vi "適應性控制_線上學習_V8(實際控制).vi"() -> ()   [LabVIEW 2010]
uses:
  <vilib>/DAQmx/read.llb/DAQmx Read (Analog 1D Wfm NChan NSamp).vi
  <vilib>/DAQmx/write.llb/DAQmx Write (Analog DBL 1Chan 1Samp).vi
  <vilib>/DAQmx/create/channels.llb/DAQmx Create Channel (AI-Voltage-Basic).vi
  <vilib>/DAQmx/configure/timing.llb/DAQmx Timing (Sample Clock).vi
  <vilib>/DAQmx/create/channels.llb/DAQmx Create Channel (AO-Voltage-Basic).vi
  <vilib>/daqmx/miscellaneous.llb/DAQmx Fill In Error Info.vi
panel:
  in  "kp":dbl
  out "理想與FIR輸出 2":dbl(graph)
  in  "模式選擇":bool=TRUE
  in  "電路 channels":tag="PXI-4472/ai1"
  in  "加速規 channels":tag="PXI-4472/ai0"
  out "輸入訊號":dbl[][](graph)
  out "輸出是否超過範圍":bool
  out "while平均執行時間(ms)":dbl
  out "Time (s)":dbl caption="Elapsed Time (s)"
  in  "error in":errorcluster
  in  "DAQ output":tag="PXI-6733/ao3"
  out "source out":string
  out "當下誤差":dbl=0.1 format="%#_13g"
  out "理想與FIR輸出":dbl[][](graph)
  out "誤差":dbl(graph)
  out "權重(w)":dbl[](array[numeric])
  in  "收斂係數":dbl=0.0001
  in  "order":i32=150
  in  "\"每\"通道取樣頻率":dbl=1000.0 min=1.0 max=10000.0 step=1.0
  in  "stop":bool
  # "版本資訊\nV6:線上學習初版\nV7:設置濾DC固定為1秒\n     新增補償擷取卡取樣與濾波器相位\nV8:修復無延遲訊號部份無濾除DC造成控制失敗\n     增加KP增益於加速規輸入讓系統自動學習增益權重"
  # "ª`·N¨Æ¶µ\n(1)ÂoDC®É­nª`·N¥­§¡¼Æ¾Úªº¸ê®Æ¼Æ,»Ý¬°±±¨î°T¸¹ÀW²vªº¾ã­Ó¶g´Áªº¸ê®Æ¼Æ,¹w³]¥­§¡1¬í¼Æ¾Ú,§Y¥i±±¨î¨ì1Hz°T¸¹\n(2)¦h³q¹D±Ä¼Ë®É,­ì¥»¿é¤Jªº¨ú¼ËÀW²v·|ÀH³q¹D¼Æ¦h¹è³Q¥­§¡±¼,¤H¾÷¤¶­±¬O¿é¤J\"¨C\"³q¹D¨ú¼ËÀW²v"
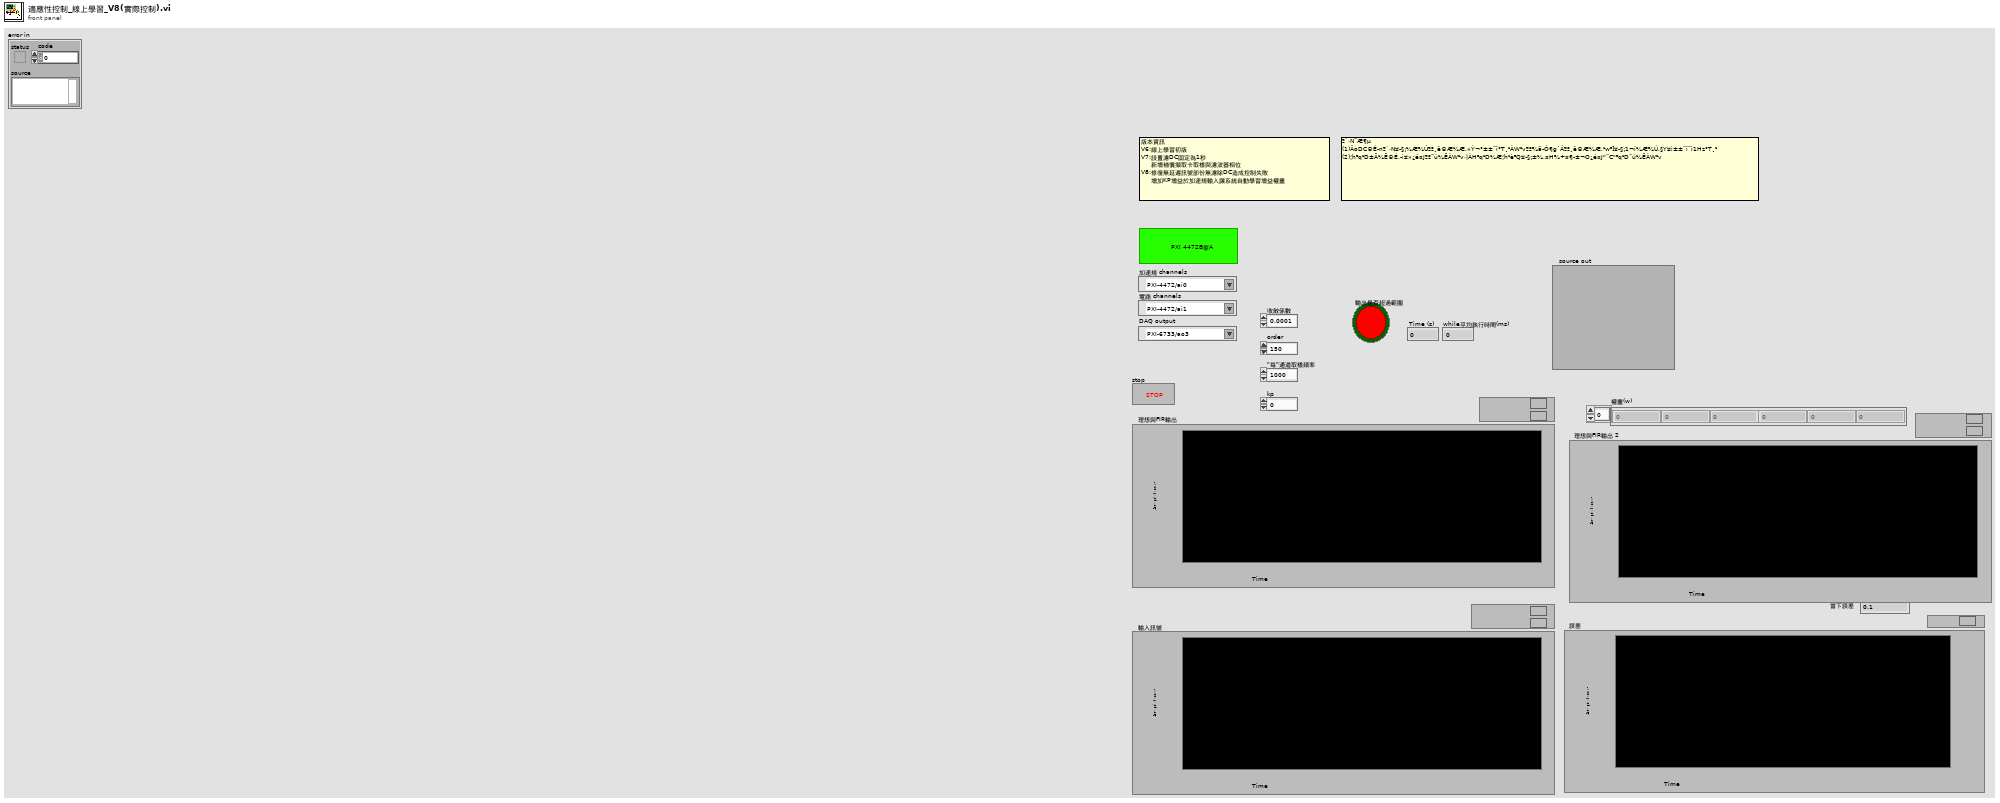
[diagram p1: front panel]
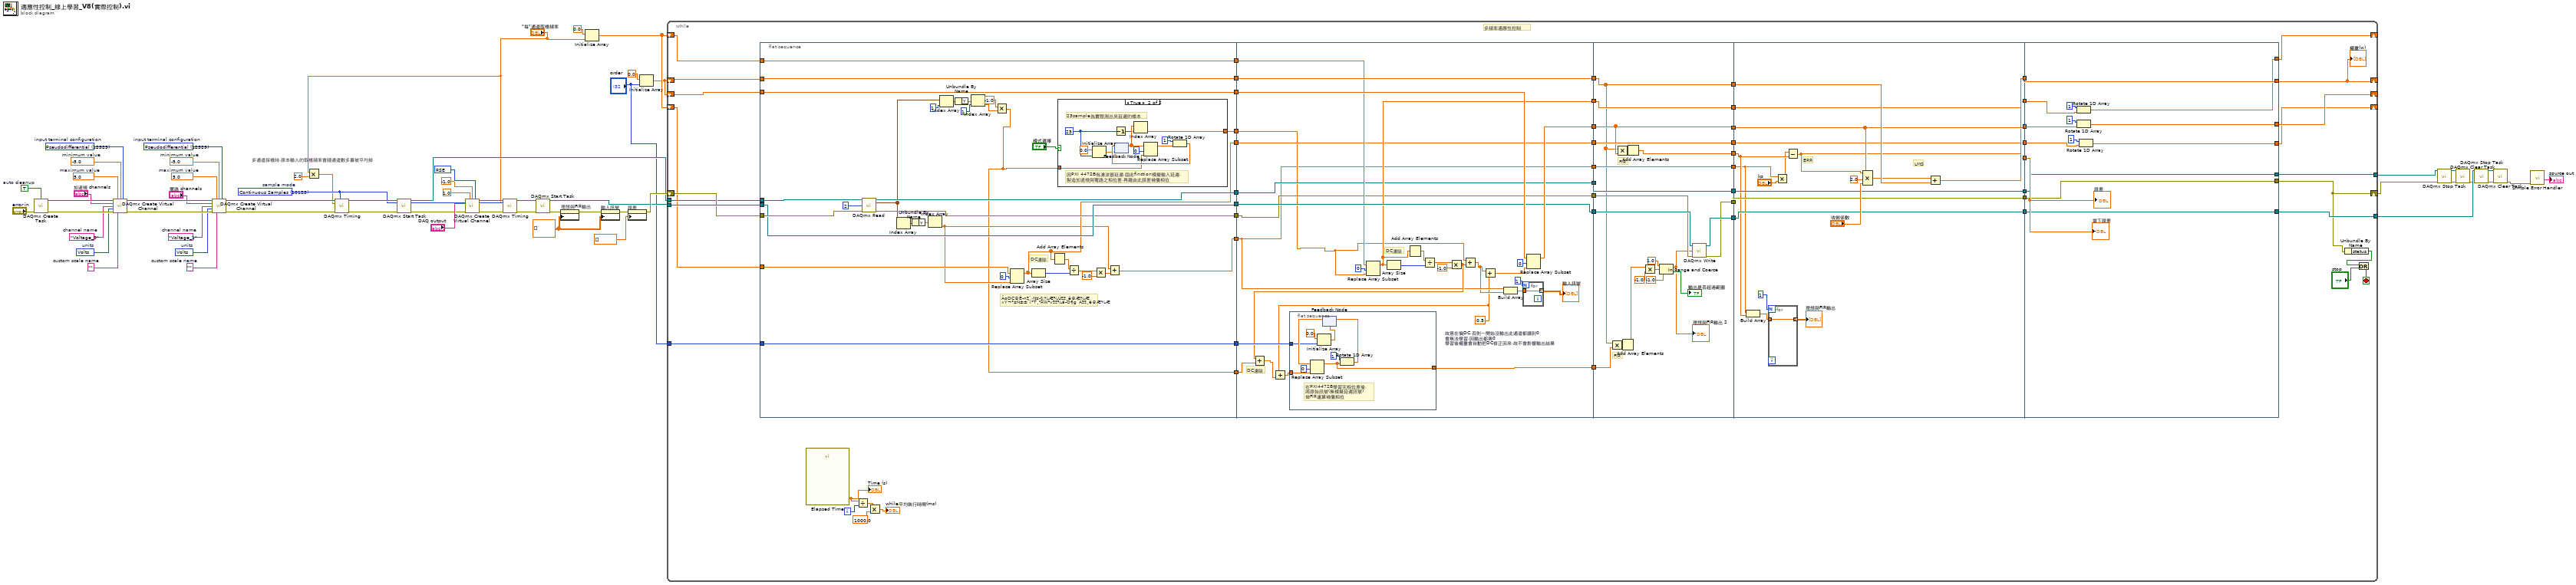
[diagram p0: block diagram]
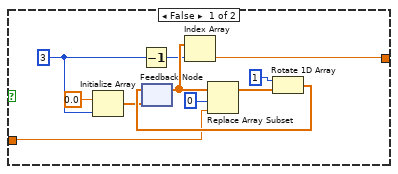
[diagram p2: hidden frame]
diagram:
  w18 = 10123 items=["Finite Samples"=10178, "Continuous Samples"=10123, "Hardware Timed Single Point"=12522]  # sample mode
  w21 = 12529 items=["default"=-1, "RSE"=10083, "NRSE"=10078, "Differential"=10106, "Pseudodifferential"=12529]  # input terminal configuration
  w22 = 10348 items=["Volts"=10348, "From Custom Scale"=10065]  # units
  w23 = "Voltage_1"  # channel name
  w25 = ""  # custom scale name
  w26 = -5.0  # minimum value
  w27 = 5.0  # maximum value
  w28 = 12529 items=["default"=-1, "RSE"=10083, "NRSE"=10078, "Differential"=10106, "Pseudodifferential"=12529]  # input terminal configuration
  w29 = 10348 items=["Volts"=10348, "From Custom Scale"=10065]  # units
  w30 = "Voltage_0"  # channel name
  w32 = ""  # custom scale name
  w33 = -5.0  # minimum value
  w34 = 5.0  # maximum value
  w36 = TRUE  # auto cleanup
  w54 = 10083 items=["Default"=-1, "RSE"=10083, "Differential"=10106, "Pseudodifferential"=12529] ("output terminal configuration")
  w8 = dbl[][] [] ("History Data")
  # "多通道採樣時,原本輸入的取樣頻率會隨通道數多寡被平均掉"
  n1 = call <vilib>:"DAQmx Create Task.vi"("auto cleanup"=w36, "error in"="error in") -> ("task out"=w35:refnum<k21>, "error out"=w37:errorcluster)  [unwired: 12 in]
  n2 = call-poly <vilib>:"DAQmx Create Virtual Channel.vi"("task in"=w35, "maximum value"=w34, "minimum value"=w33, "input terminal configuration"=w28, "physical channels"="加速規 channels", "name to assign"=w30, "units"=w29, "error in"=w37, "custom scale name"=w32) -> ("task out"=w14:refnum<k21>, "error out"=w31:errorcluster)  [unwired: 5 in]
  n3 = call-poly <vilib>:"DAQmx Create Virtual Channel.vi"("task in"=w14, "maximum value"=w27, "minimum value"=w26, "input terminal configuration"=w21, "physical channels"="電路 channels", "name to assign"=w23, "units"=w22, "error in"=w31, "custom scale name"=w25) -> ("task out"=w20:refnum<k21>, "error out"=w24:errorcluster)  [unwired: 5 in]
  n4 = Multiply(x="\"每\"通道取樣頻率", y=2.0) -> (x*y=w5:dbl)
  n5 = call-poly <vilib>:"DAQmx Timing.vi"("task/channels in"=w20, "sample mode"=w18, "rate"=w5, "error in"=w24) -> ("task out"=w19:refnum<k21>, "error out"=w15:errorcluster)  [unwired: 10 in]
  n6 = call <vilib>:"DAQmx Start Task.vi"("task/channels in"=w19, "error in"=w15) -> ("task out"=w16:refnum<k21>, "error out"=w42:errorcluster)  [unwired: 12 in]
  n7 = call-poly <vilib>:"DAQmx Create Virtual Channel.vi"("maximum value"=1.0, "minimum value"=-1.0, "output terminal configuration"=w54, "physical channels"="DAQ output", "error in"=w42) -> ("task out"=w55:refnum<k21>, "error out"=w58:errorcluster)  [unwired: 9 in]
  n8 = call-poly <vilib>:"DAQmx Timing.vi"("task/channels in"=w55, "sample mode"=w18, "rate"="\"每\"通道取樣頻率", "error in"=w58) -> ("task out"=w56:refnum<k21>, "error out"=w57:errorcluster)  [unwired: 10 in]
  n9 = call <vilib>:"DAQmx Start Task.vi"("task/channels in"=w56, "error in"=w57) -> ("task out"=w12:refnum<k21>, "error out"=w17:errorcluster)  [unwired: 12 in]
  n10 = property on="理想與FIR輸出" class="WFChart (strict)"(error in=w17, "History Data"=w8) -> (error out=w10:errorcluster)  [unwired: 1 in, 1 out]
  n11 = Initialize Array(0.0 ("element"), "\"每\"通道取樣頻率") -> (w4:dbl[])
  n12 = property on="輸入訊號" class="WFChart (strict)"(error in=w10, "History Data"=w8) -> (error out=w9:errorcluster)  [unwired: 1 in, 1 out]
  n13 = property on="誤差" class="WFChart (strict)"(error in=w9, "History Data"=dbl[] []) -> (error out=w40:errorcluster)  [unwired: 1 in, 1 out]
  n14 = Initialize Array(0.0 ("element"), "order") -> (w3:dbl[])
  n15 = while {
    shift-right: [w107] -> _
    shift-left: w3 -> [w119]
    shift-right: [w111] -> _
    shift-left: w3 -> [w115]
    tunnel: w12 -> [w106]
    tunnel: [w92] -> w49
    tunnel: [w91] -> w48
    shift-right: [w78] -> _
    shift-left: w4 -> [w88]
    tunnel: w16 -> [w80]
    shift-right: [w79] -> w13
    shift-left: w40 -> [w105]
    shift-right: [w71] -> _
    shift-left: w4 -> [w72]
    tunnel: "order" -> [w62]
    i -> [w66]
    stop <- w89 stop-if-true
    # "多頻率適應性控制"
    n16 = flat-sequence {
      tunnel: [w152] -> w120
      tunnel: w119 -> [w152]
      tunnel: [w151] -> w116
      tunnel: w115 -> [w151]
      tunnel: w106 -> [w139]
      tunnel: w105 -> [w149]
      tunnel: [w148] -> w104
      tunnel: [w138] -> w103
      tunnel: [w139] -> w96
      tunnel: w88 -> [w150]
      tunnel: [w150] -> w87
      tunnel: w80 -> [w141]
      tunnel: [w121] -> w77
      tunnel: w72 -> [w131]
      tunnel: [w130] -> w67
      tunnel: [w122] -> w65
      tunnel: w62 -> [w127]
      tunnel: [w127] -> w63
      tunnel: [w125] -> w61
      tunnel: w120 -> [w201]
      tunnel: [w203] -> w118
      tunnel: [w202] -> w117
      tunnel: w116 -> [w202]
      tunnel: w104 -> [w192]
      tunnel: w103 -> [w191]
      tunnel: [w191] -> w102
      tunnel: [w192] -> w99
      tunnel: [w200] -> w97
      tunnel: w96 -> [w200]
      tunnel: w87 -> [w195]
      tunnel: [w194] -> w86
      tunnel: [w180] -> w81
      tunnel: w77 -> [w180]
      tunnel: [w188] -> w68
      tunnel: w67 -> [w188]
      tunnel: w65 -> [w182]
      tunnel: [w185] -> w64
      tunnel: w63 -> [w184]
      tunnel: w61 -> [w183]
      tunnel: w118 -> [w220]
      tunnel: w117 -> [w217]
      tunnel: [w217] -> w114
      tunnel: [w215] -> w113
      tunnel: [w220] -> w112
      tunnel: w102 -> [w222]
      tunnel: [w221] -> w101
      tunnel: w99 -> [w233]
      tunnel: [w233] -> w98
      tunnel: w97 -> [w226]
      tunnel: [w225] -> w95
      tunnel: w86 -> [w232]
      tunnel: [w232] -> w85
      tunnel: [w231] -> w82
      tunnel: w81 -> [w231]
      tunnel: [w224] -> w69
      tunnel: w68 -> [w224]
      tunnel: w64 -> [w218]
      tunnel: w114 -> [w253]
      tunnel: w113 -> [w238]
      tunnel: w112 -> [w249]
      tunnel: [w247] -> w110
      tunnel: [w249] -> w109
      tunnel: [w242] -> w108
      tunnel: w101 -> [w246]
      tunnel: [w246] -> w100
      tunnel: w98 -> [w245]
      tunnel: w95 -> [w241]
      tunnel: [w241] -> w94
      tunnel: [w245] -> w93
      tunnel: w85 -> [w244]
      tunnel: [w244] -> w84
      tunnel: w82 -> [w236]
      tunnel: [w239] -> w70
      tunnel: w69 -> [w239]
      tunnel: [w268] -> w111
      tunnel: w110 -> [w268]
      tunnel: w109 -> [w265]
      tunnel: [w267] -> w107
      tunnel: w108 -> [w264]
      tunnel: w100 -> [w263]
      tunnel: [w263] -> w79
      tunnel: w94 -> [w261]
      tunnel: w93 -> [w262]
      tunnel: [w262] -> w92
      tunnel: [w261] -> w91
      tunnel: [w258] -> w78
      tunnel: w84 -> [w259]
      tunnel: [w256] -> w71
      tunnel: w70 -> [w255]
      frame #0 {
        # "ÂoDC®É­nª`·N¥­§¡¼Æ¾Úªº¸ê®Æ¼Æ\n»Ý¬°¥N±±¨î°T¸¹ÀW²vªº¾ã­Ó¶g´Áªº¸ê®Æ¼Æ"
        # "DC濾除"
        n17 = call-poly <vilib>:"DAQmx Read.vi"("task/channels in"=w141, "number of samples per channel"=2, "error in"=w149) -> ("task out"=w148:refnum<k21>, "data"=w142:waveform(dbl)[], "error out"=w138:errorcluster)  [unwired: 10 in]
        n18 = Index Array(array=w142) -> (element=w147:waveform(dbl))  [unwired: 1 in]
        n19 = Unbundle By Name(w147) -> ("Y"=w146:dbl[])
        n20 = Index Array(array=w146) -> (element=w129:dbl)  [unwired: 1 in]
        n21 = Index Array(array=w142, index=1) -> (element=w145:waveform(dbl))
        n22 = Unbundle By Name(w145) -> ("Y"=w144:dbl[])
        n23 = Index Array(array=w144, index=1) -> (element=w124:dbl)
        n24 = Multiply(x=-1.0, y=w124) -> (x*y=w122:dbl)
        n25 = Replace Array Subset(array=w131, new element=w129, index=0) -> (w130:dbl[])
        n26 = Array Size(array=w130) -> (size(s)=w135:i32)
        n27 = Add Array Elements(numeric array=w130) -> (sum=w134:dbl)
        n28 = case shown="True" "模式選擇" {
          tunnel: [w153 w171] -> w125
          tunnel: w122 -> [w154 w168]
          frame False {
            w155 = 3 ("index")
            n29 = Initialize Array(0.0 ("element"), w155) -> (w157:dbl[])
            n30 = Decrement(x=w155) -> (x-1=w156:i32)
            n31 = feedback #1(w157) -> (w159:dbl[])
            n32 = Index Array(array=w159, index=w156) -> (element=w153:dbl)
            n33 = Replace Array Subset(array=w159, new element=w154, index=0) -> (w162:dbl[])
            n34 = Rotate 1D Array(1:w162, 2:1 ("n")) -> (0:w160:dbl[])
            n35 = feedback-in #1(w160) -> ()
          }
          frame True {
            w164 = 23 ("index")
            # "23sample為實際測出來延遲的樣本"
            # "因PXI 4472B有濾波器延遲,固此finction模擬輸入延遲,\n製造加速規與電路之相位差,再藉由此誤差補償相位"
            n36 = Initialize Array(0.0 ("element"), w164) -> (w166:dbl[])
            n37 = Decrement(x=w164) -> (x-1=w165:i32)
            n38 = feedback #2(w166) -> (w169:dbl[])
            n39 = Index Array(array=w169, index=w165) -> (element=w171:dbl)
            n40 = Replace Array Subset(array=w169, new element=w168, index=0) -> (w173:dbl[])
            n41 = Rotate 1D Array(1:w173, 2:1 ("n")) -> (0:w170:dbl[])
            n42 = feedback-in #2(w170) -> ()
          }
        }
        n43 = Divide(x=w134, y=w135) -> (x/y=w136:dbl)
        n44 = Multiply(x=w136, y=-1.0) -> (x*y=w137:dbl)
        n45 = Add(x=w129, y=w137) -> (x+y=w121:dbl)
      }
      frame #1 {
        w176 = 0.5  # 故意在偏DC,否則一開始沒輸出此通道都讀到0 會無法學習,因輸出都乘0 學習後權重會自動把DC修正回來,故不會影響輸出結果
        # "DC濾除"
        # "DC濾除"
        n46 = flat-sequence {
          tunnel: w177 -> [w211]
          tunnel: [w205] -> w185
          tunnel: w184 -> [w204]
          frame #0 {
            # "在PXI4472B學習完相位差後,\n將原始訊號(無模擬延遲訊號)\n做FIR運算補償相位"
            n47 = Initialize Array(0.0 ("element"), w204) -> (w207:dbl[])
            n48 = feedback #3(w207) -> (w209:dbl[])
            n49 = Replace Array Subset(array=w209, new element=w211, index=0) -> (w205:dbl[])
            n50 = Rotate 1D Array(1:w205, 2:1 ("n")) -> (0:w210:dbl[])
            n51 = feedback-in #3(w210) -> ()
          }
        }
        n52 = Replace Array Subset(array=w195, new element=w183, index=0) -> (w194:dbl[])
        n53 = Array Size(array=w194) -> (size(s)=w198:i32)
        n54 = Add Array Elements(numeric array=w194) -> (sum=w197:dbl)
        n55 = Divide(x=w197, y=w198) -> (x/y=w199:dbl)
        n56 = Multiply(x=w199, y=-1.0) -> (x*y=w181:dbl)
        n57 = Add(x=w181, y=w182) -> (x+y=w175:dbl)
        n58 = Add(x=w176, y=w175) -> (x+y=w177:dbl)
        n59 = Add(x=w183, y=w181) -> (x+y=w179:dbl)
        n60 = Add(x=w179, y=w176) -> (x+y=w178:dbl)
        n61 = Build Array(w180, w179) -> (w190:dbl[])
        n62 = for {
          N: 1 -> [_]
          tunnel: w190 -> [w213]
          tunnel: [w213] -> w187 mode=indexing
        }
        "輸入訊號" <- w187
        n63 = Replace Array Subset(array=w201, new element=w178, index=0) -> (w203:dbl[])
      }
      frame #2 {
        # "FIR"
        # "FIR"
        n64 = Multiply(x=w217, y=w218) -> (x*y=w219:dbl[])
        n65 = Multiply(x=w217, y=w220) -> (x*y=w234:dbl[])
        n66 = Add Array Elements(numeric array=w219) -> (sum=w216:dbl)
        n67 = Add Array Elements(numeric array=w234) -> (sum=w215:dbl)
        n68 = Multiply(x=w216, y=-1.0) -> (x*y=w229:dbl)
        n69 = In Range and Coerce(upper limit=1.0, x=w229, lower limit=-1.0 ("upper limit")) -> (coerced(x)=w214:dbl, In Range?=→"輸出是否超過範圍":bool)
        "理想與FIR輸出 2" <- w214
        n70 = call-poly <vilib>:"DAQmx Write.vi"("task/channels in"=w226, "data"=w214, "error in"=w222) -> ("task out"=w225:refnum<k21>, "error out"=w221:errorcluster)  [unwired: 10 in, 1 out]
      }
      frame #3 {
        # "LMS"
        # "ERR"
        n71 = Build Array(w236, w238) -> (w252:dbl[])
        n72 = for {
          N: 1 -> [_]
          tunnel: [w254] -> w240 mode=indexing
          tunnel: w252 -> [w254]
        }
        "理想與FIR輸出" <- w240
        n73 = Multiply(x=w236, y="kp") -> (x*y=w235:dbl)
        n74 = Subtract(x=w235, y=w238) -> (x-y=w242:dbl)
        n75 = Compound Arithmetic op=MULTIPLY(w242, w249, 2.0, "收斂係數") -> (w248:dbl[])
        n76 = Add(x=w248, y=w253) -> (x+y=w247:dbl[])
      }
      frame #4 {
        n77 = Rotate 1D Array(1:w259, 2:1 ("n")) -> (0:w258:dbl[])
        n78 = Rotate 1D Array(1:w265, 2:1 ("n")) -> (0:w267:dbl[])
        n79 = Rotate 1D Array(1:w255, 2:1 ("n")) -> (0:w256:dbl[])
        "誤差" <- w264
        "當下誤差" <- w264
      }
    }
    n80 = call "Elapsed Time"() -> ("Elapsed Time (s)"=w76:dbl)  [unwired: 12 in, 7 out]
    "Time (s)" <- w76
    n81 = Divide(x=w76, y=w66) -> (x/y=w75:dbl)
    n82 = Multiply(x=w75, y=1000.0) -> (x*y=→"while平均執行時間(ms)":dbl)
    n83 = Unbundle By Name(w79) -> ("status"=w83:bool)
    n84 = Or(x=w83, y="stop") -> (x .or. y?=w89:bool)
    "權重(w)" <- w111
  }
  n85 = call <vilib>:"DAQmx Stop Task.vi"("task/channels in"=w49, "error in"=w13) -> ("task out"=w51:refnum<k21>, "error out"=w50:errorcluster)  [unwired: 12 in]
  n86 = call <vilib>:"DAQmx Clear Task.vi"("task in"=w51, "error in"=w50) -> ("error out"=w41:errorcluster)  [unwired: 13 in]
  n87 = call <vilib>:"DAQmx Stop Task.vi"("task/channels in"=w48, "error in"=w41) -> ("task out"=w46:refnum<k21>, "error out"=w47:errorcluster)  [unwired: 12 in]
  n88 = call <vilib>:"DAQmx Clear Task.vi"("task in"=w46, "error in"=w47) -> ("error out"=w39:errorcluster)  [unwired: 13 in]
  n89 = call <vilib>:"Simple Error Handler.vi"("error in (no error)"=w39) -> ("source out"=→"source out":string)  [unwired: 4 in, 4 out]
